vi "OpenAvi.vi"(11 "camera":u64) -> (3 "aviFile out":T1)   [LabVIEW 2019]
uses:
  EmergentCameraC/EmergentCameraC.lvlib
panel:
  in  "aviFile":T1
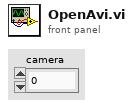
[diagram p1: front panel]
types:
  T1 = cluster{"fileName[0]":i8, "fileName[1]":i8, "fileName[2]":i8, "fileName[3]":i8, "fileName[4]":i8, "fileName[5]":i8, "fileName[6]":i8, "fileName[7]":i8, "fileName[8]":i8, "fileName[9]":i8, "fileName[10]":i8, "fileName[11]":i8, "fileName[12]":i8, "fileName[13]":i8, "fileName[14]":i8, "fileName[15]":i8, "fileName[16]":i8, "fileName[17]":i8, "fileName[18]":i8, "fileName[19]":i8, "fileName[20]":i8, "fileName[21]":i8, "fileName[22]":i8, "fileName[23]":i8, "fileName[24]":i8, "fileName[25]":i8, "fileName[26]":i8, "fileName[27]":i8, "fileName[28]":i8, "fileName[29]":i8, "fileName[30]":i8, "fileName[31]":i8, "fileName[32]":i8, "fileName[33]":i8, "fileName[34]":i8, "fileName[35]":i8, "fileName[36]":i8, "fileName[37]":i8, "fileName[38]":i8, "fileName[39]":i8, "fileName[40]":i8, "fileName[41]":i8, "fileName[42]":i8, "fileName[43]":i8, "fileName[44]":i8, "fileName[45]":i8, "fileName[46]":i8, "fileName[47]":i8, "fileName[48]":i8, "fileName[49]":i8, "fileName[50]":i8, "fileName[51]":i8, "fileName[52]":i8, "fileName[53]":i8, "fileName[54]":i8, "fileName[55]":i8, "fileName[56]":i8, "fileName[57]":i8, "fileName[58]":i8, "fileName[59]":i8, "fileName[60]":i8, "fileName[61]":i8, "fileName[62]":i8, "fileName[63]":i8, "fileName[64]":i8, "fileName[65]":i8, "fileName[66]":i8, "fileName[67]":i8, "fileName[68]":i8, "fileName[69]":i8, "fileName[70]":i8, "fileName[71]":i8, "fileName[72]":i8, "fileName[73]":i8, "fileName[74]":i8, "fileName[75]":i8, "fileName[76]":i8, "fileName[77]":i8, "fileName[78]":i8, "fileName[79]":i8, "fileName[80]":i8, "fileName[81]":i8, "fileName[82]":i8, "fileName[83]":i8, "fileName[84]":i8, "fileName[85]":i8, "fileName[86]":i8, "fileName[87]":i8, "fileName[88]":i8, "fileName[89]":i8, "fileName[90]":i8, "fileName[91]":i8, "fileName[92]":i8, "fileName[93]":i8, "fileName[94]":i8, "fileName[95]":i8, "fileName[96]":i8, "fileName[97]":i8, "fileName[98]":i8, "fileName[99]":i8, "fileName[100]":i8, "fileName[101]":i8, "fileName[102]":i8, "fileName[103]":i8, "fileName[104]":i8, "fileName[105]":i8, "fileName[106]":i8, "fileName[107]":i8, "fileName[108]":i8, "fileName[109]":i8, "fileName[110]":i8, "fileName[111]":i8, "fileName[112]":i8, "fileName[113]":i8, "fileName[114]":i8, "fileName[115]":i8, "fileName[116]":i8, "fileName[117]":i8, "fileName[118]":i8, "fileName[119]":i8, "fileName[120]":i8, "fileName[121]":i8, "fileName[122]":i8, "fileName[123]":i8, "fileName[124]":i8, "fileName[125]":i8, "fileName[126]":i8, "fileName[127]":i8, "fileName[128]":i8, "fileName[129]":i8, "fileName[130]":i8, "fileName[131]":i8, "fileName[132]":i8, "fileName[133]":i8, "fileName[134]":i8, "fileName[135]":i8, "fileName[136]":i8, "fileName[137]":i8, "fileName[138]":i8, "fileName[139]":i8, "fileName[140]":i8, "fileName[141]":i8, "fileName[142]":i8, "fileName[143]":i8, "fileName[144]":i8, "fileName[145]":i8, "fileName[146]":i8, "fileName[147]":i8, "fileName[148]":i8, "fileName[149]":i8, "fileName[150]":i8, "fileName[151]":i8, "fileName[152]":i8, "fileName[153]":i8, "fileName[154]":i8, "fileName[155]":i8, "fileName[156]":i8, "fileName[157]":i8, "fileName[158]":i8, "fileName[159]":i8, "fileName[160]":i8, "fileName[161]":i8, "fileName[162]":i8, "fileName[163]":i8, "fileName[164]":i8, "fileName[165]":i8, "fileName[166]":i8, "fileName[167]":i8, "fileName[168]":i8, "fileName[169]":i8, "fileName[170]":i8, "fileName[171]":i8, "fileName[172]":i8, "fileName[173]":i8, "fileName[174]":i8, "fileName[175]":i8, "fileName[176]":i8, "fileName[177]":i8, "fileName[178]":i8, "fileName[179]":i8, "fileName[180]":i8, "fileName[181]":i8, "fileName[182]":i8, "fileName[183]":i8, "fileName[184]":i8, "fileName[185]":i8, "fileName[186]":i8, "fileName[187]":i8, "fileName[188]":i8, "fileName[189]":i8, "fileName[190]":i8, "fileName[191]":i8, "fileName[192]":i8, "fileName[193]":i8, "fileName[194]":i8, "fileName[195]":i8, "fileName[196]":i8, "fileName[197]":i8, "fileName[198]":i8, "fileName[199]":i8, "fileName[200]":i8, "fileName[201]":i8, "fileName[202]":i8, "fileName[203]":i8, "fileName[204]":i8, "fileName[205]":i8, "fileName[206]":i8, "fileName[207]":i8, "fileName[208]":i8, "fileName[209]":i8, "fileName[210]":i8, "fileName[211]":i8, "fileName[212]":i8, "fileName[213]":i8, "fileName[214]":i8, "fileName[215]":i8, "fileName[216]":i8, "fileName[217]":i8, "fileName[218]":i8, "fileName[219]":i8, "fileName[220]":i8, "fileName[221]":i8, "fileName[222]":i8, "fileName[223]":i8, "fileName[224]":i8, "fileName[225]":i8, "fileName[226]":i8, "fileName[227]":i8, "fileName[228]":i8, "fileName[229]":i8, "fileName[230]":i8, "fileName[231]":i8, "fileName[232]":i8, "fileName[233]":i8, "fileName[234]":i8, "fileName[235]":i8, "fileName[236]":i8, "fileName[237]":i8, "fileName[238]":i8, "fileName[239]":i8, "fileName[240]":i8, "fileName[241]":i8, "fileName[242]":i8, "fileName[243]":i8, "fileName[244]":i8, "fileName[245]":i8, "fileName[246]":i8, "fileName[247]":i8, "fileName[248]":i8, "fileName[249]":i8, "fileName[250]":i8, "fileName[251]":i8, "fileName[252]":i8, "fileName[253]":i8, "fileName[254]":i8, "fileName[255]":i8, "codec":i32, "@dummy control@":i8, "@dummy control@":i8, "@dummy control@":i8, "@dummy control@":i8, "fps":dbl, "width":i32, "height":i32, "isColor":i32, "@dummy control@":i8, "@dummy control@":i8, "@dummy control@":i8, "@dummy control@":i8, "privateData":i64}
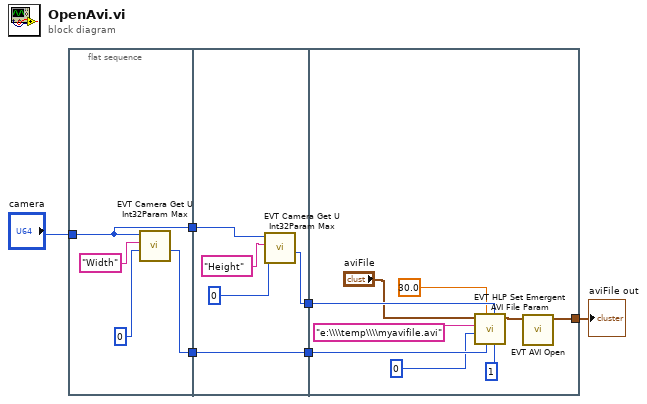
[diagram p0: block diagram]
diagram:
  n1 = flat-sequence {
    tunnel: "camera" -> [w9]
    tunnel: [w9] -> w6
    tunnel: [w7] -> w3
    tunnel: w6 -> [w12]
    tunnel: [w13] -> w4
    tunnel: w3 -> [w11]
    tunnel: [w11] -> w2
    tunnel: w4 -> [w24]
    tunnel: w2 -> [w23]
    tunnel: [w16] -> w1
    frame #0 {
      n2 = call "EVT Camera Get U Int32Param Max.vi"("max"=u32 0, "name"="Width", "camera"=w9) -> ("max out"=w7:u32)  [unwired: 7 in, 1 out]
    }
    frame #1 {
      n3 = call "EVT Camera Get U Int32Param Max.vi"("max"=u32 0, "name"="Height", "camera"=w12) -> ("max out"=w13:u32)  [unwired: 7 in, 1 out]
    }
    frame #2 {
      n4 = call "EVT HLP Set Emergent AVI File Param.vi"("isColor"=1, "height"=w24, "width"=w23, "fps"=30.0, "codec"=0, "fileName"="e:\\\\temp\\\\myavifile.avi", "aviFile"="aviFile") -> ("aviFile out"=w18:T1)  [unwired: 3 in, 1 out]
      n5 = call "EVT AVI Open.vi"("aviFile"=w18) -> ("aviFile out"=w16:T1)  [unwired: 9 in, 1 out]
    }
  }
  "aviFile out" <- w1
